vi "TimeTEST.vi"(8 "VISA resource name":refnum<visa-resource-name>, 9 "relative seconds":dbl format="%_19f") -> (0 "VISA resource name 2":refnum<visa-resource-name>, 2 "New Time":dbl format="%_19f", 3 "Delta":dbl)   [LabVIEW 2021]
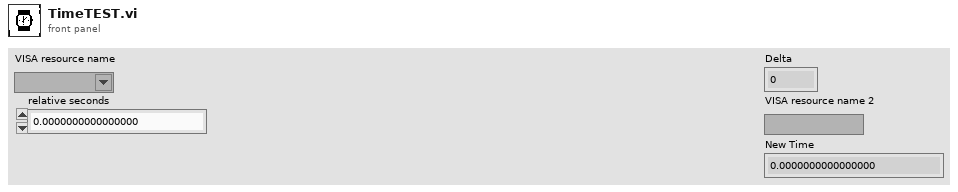
[diagram p1: front panel]
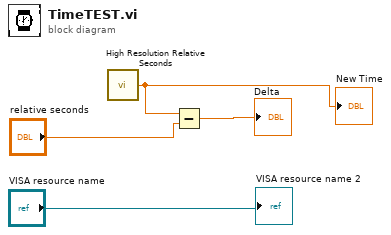
[diagram p0: block diagram]
diagram:
  n1 = call <vilib>:"High Resolution Relative Seconds.vi"() -> ("relative seconds"=w4:dbl)
  "New Time" <- w4
  n2 = Subtract(x=w4, y="relative seconds") -> (x-y=→"Delta":dbl)
  "VISA resource name 2" <- "VISA resource name"
